vi "PH_BL-Master.get 6P 4Q Position by Name.vi"(0 "i ref in":refnum<vi>, 2 "6P 4Q Instance":T1="N/A", 5 "error in (no error)":errorcluster) -> (9 "index of element":i32, 10 "Pic GUI Ref":refnum<vi>, 11 "no Link?":bool, 13 "Instance found?":bool, 14 "i ref out":refnum<vi>, 17 "Position":T2 items=["unknown", "Position I", "Position II", "Position III", "Position IV", "moving"], 19 "error out":errorcluster)   [LabVIEW 2014, in "PH_BL-Master.lvlib"]
doc: "This VI gets the position of the selected 6P 4Q Instance."
uses:
  PH_BL-Master.lvlib
  PH_Motion/PH_4_Pos_Selector/PH_4_Pos_Selector.Position Selector.ctl
  PH_Beamline/PH_Beamline.6P 4 Pos Selector Instances.ctl
  PH_Motion/PH_4_Pos_Selector/PH_4_Pos_Selector.lvlib
  PH_Beamline/PH_Beamline.lvlib
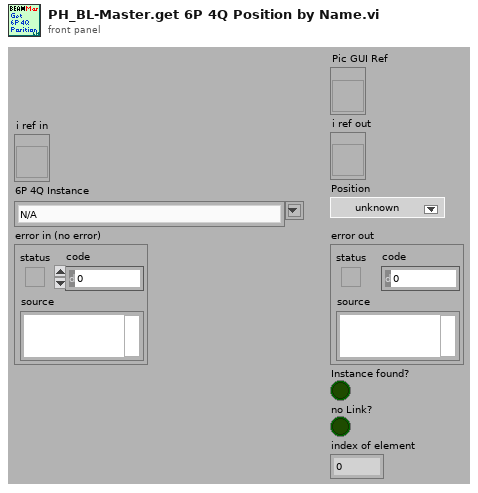
[diagram p1: front panel]
types:
  T1 = typedef "PH_Beamline.lvlib/PH_Beamline.6P 4 Pos Selector Instances.ctl" = string
  T2 = typedef "PH_4_Pos_Selector.lvlib/PH_4_Pos_Selector.Position Selector.ctl" = u16
  T3 = typedef "PH_BL-Master.lvlib/PH_BL-Master.i attribute.ctl" = cluster{"Remote controlled":bool, "Boolean Condition Service Subscriber":refnum<vi>[], "Picture Condition Service Subscriber":refnum<vi>[], "R2S":cluster{"GUI Ref":refnum<vi>, "State":bool}, "Vacua":cluster{"GUI Ref":refnum<vi>, "Limit":dbl, "Curr Value":dbl, "in range":bool}[], "O2 Inspection":cluster{"GUI Ref":refnum<vi>, "Concentration":dbl, "State":T4}[], "Boolean Status Service Subscriber":cluster{"GUI Ref":refnum<vi>, "Status":T4, "no Link?":bool, "Status Subscriber Class":T5}[], "Picture Status Service Subscriber":cluster{"GUI Ref":refnum<vi>, "Status":T4, "no Link?":bool, "Status Subscriber Class":T5}[], "6P 4Q Service Subscriber":cluster{"GUI Ref":refnum<vi>, "Selector":T2, "no Link?":bool}[], "Index of latest 6P 4Q changing Instance":i32, "Index of latest Picture Status changing Instance":i32, "Index of latest Boolean Status changing Instance":i32, "Vision ID on same Node":string, "Start Phase over?":bool, "GUI Ref Delete":refnum<vi>}
  T4 = typedef "PH_StatusHandler.lvlib/PH_StatusHandler.Status.ctl" = i16
  T5 = typedef "PH_BL-Master.lvlib/PH_BL-Master.Status Subscriber Class.ctl" = enum16{"unknown", "Switch", "BB", "6P Switch", "Switch GUI", "Switch and 6P State", "Force Sensor"}
  T6 = cluster{"GUI Ref":refnum<vi>, "Selector":T2, "no Link?":bool}[]
  T7 = cluster{"GUI Ref":refnum<vi>, "Selector":T2, "no Link?":bool}
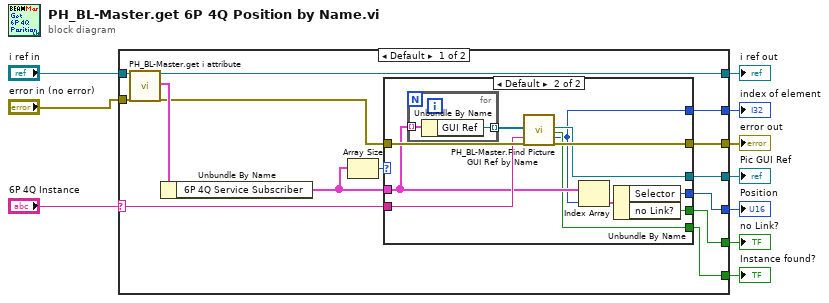
[diagram p0: block diagram]
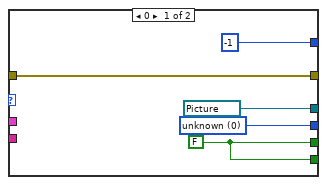
[diagram p2: hidden frame]
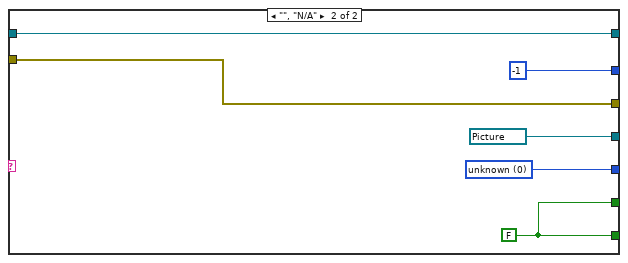
[diagram p3: hidden frame]
diagram:
  n1 = case shown="Default" "6P 4Q Instance" {
    selector: "6P 4Q Instance" -> [w18 _]
    tunnel: "error in (no error)" -> [w23 w47]
    tunnel: "i ref in" -> [w22 w48]
    tunnel: [w21 w48] -> w5
    tunnel: [w14 w46] -> w7
    tunnel: [w20 w47] -> w6
    tunnel: [w11 w45] -> w4
    tunnel: [w19 w45] -> w3
    tunnel: [w16 refnum<vi> refnum ("Wanted Pic GUI Ref")] -> w2
    tunnel: [w15 -1 ("index of element")] -> w1
    frame Default {
      n2 = call "PH_BL-Master.get i attribute.vi"("i ref in"=w22, "error in (no error)"=w23) -> ("i ref out"=w21:refnum<vi>, "i attribute"=w24:T3, "error out"=w13:errorcluster)  [unwired: 15 in]
      n3 = Unbundle By Name(w24) -> ("6P 4Q Service Subscriber"=w17:T6)
      n4 = Array Size(array=w17) -> (size(s)=w12:i32)
      n5 = case shown="Default" w12 {
        tunnel: w17 -> [_ w36]
        tunnel: w18 -> [_ w38]
        tunnel: [w29 w37] -> w20
        tunnel: [w28 w33] -> w14
        tunnel: w13 -> [w29 w39]
        tunnel: [w27 w32] -> w11
        tunnel: [w27 w34] -> w19
        tunnel: [refnum<vi> refnum ("Wanted Pic GUI Ref") w31] -> w16
        tunnel: [-1 ("index of element") w30] -> w15
        frame 0 {
          w27 = FALSE
          w28 = T2 0 items=["unknown", "Position I", "Position II", "Position III", "Position IV", "moving"] ("State")
        }
        frame Default {
          n6 = for {
            tunnel: w36 -> [w42] mode=indexing
            tunnel: [w41] -> w40 mode=indexing
            n7 = Unbundle By Name(w42) -> ("GUI Ref"=w41:refnum<vi>)
          }
          n8 = call "PH_BL-Master.Find Picture GUI Ref by Name.vi"("Pic Ref Array"=w40, "Label"=w38, "error in"=w39) -> ("Wanted Pic GUI Ref"=w31:refnum<vi>, "Ref found?"=w32:bool, "index of element"=w30:i32, "error out"=w37:errorcluster)  [unwired: 13 in]
          n9 = Index Array(array=w36, index=w30) -> (element=w35:T7)
          n10 = Unbundle By Name(w35) -> ("Selector"=w33:T2, "no Link?"=w34:bool)
        }
      }
    }
    frame "", "N/A" {
      w45 = FALSE
      w46 = T2 0 items=["unknown", "Position I", "Position II", "Position III", "Position IV", "moving"] ("State")
    }
  }
  "i ref out" <- w5
  "error out" <- w6
  "Position" <- w7
  "Instance found?" <- w4
  "no Link?" <- w3
  "Pic GUI Ref" <- w2
  "index of element" <- w1
